vi "Calcul itératif.vi"(10 "Température capteur 1-2-3-4-Ambiant":dbl[](array[numeric]), 11 "Position des capteurs":dbl[][](array[numeric])) -> (3 "DATA - T/R1/R2/R3":dbl[](array[numeric]) format="%#_13g")   [LabVIEW 2018]
panel:
  in  "T max":dbl
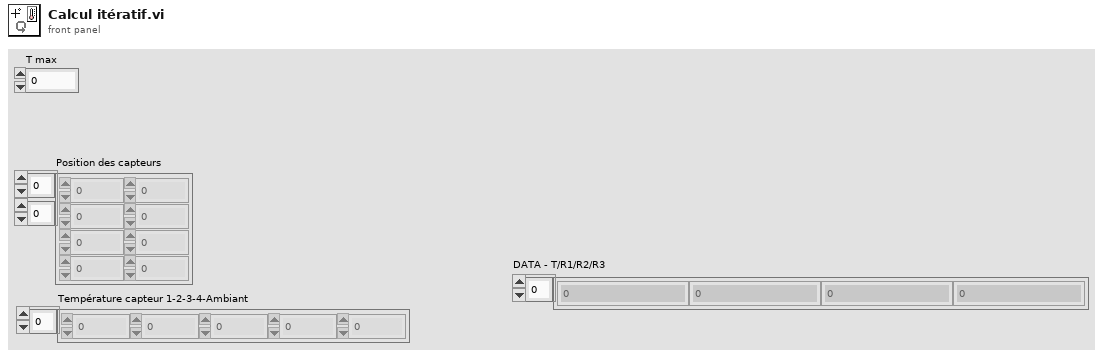
[diagram p1: front panel]
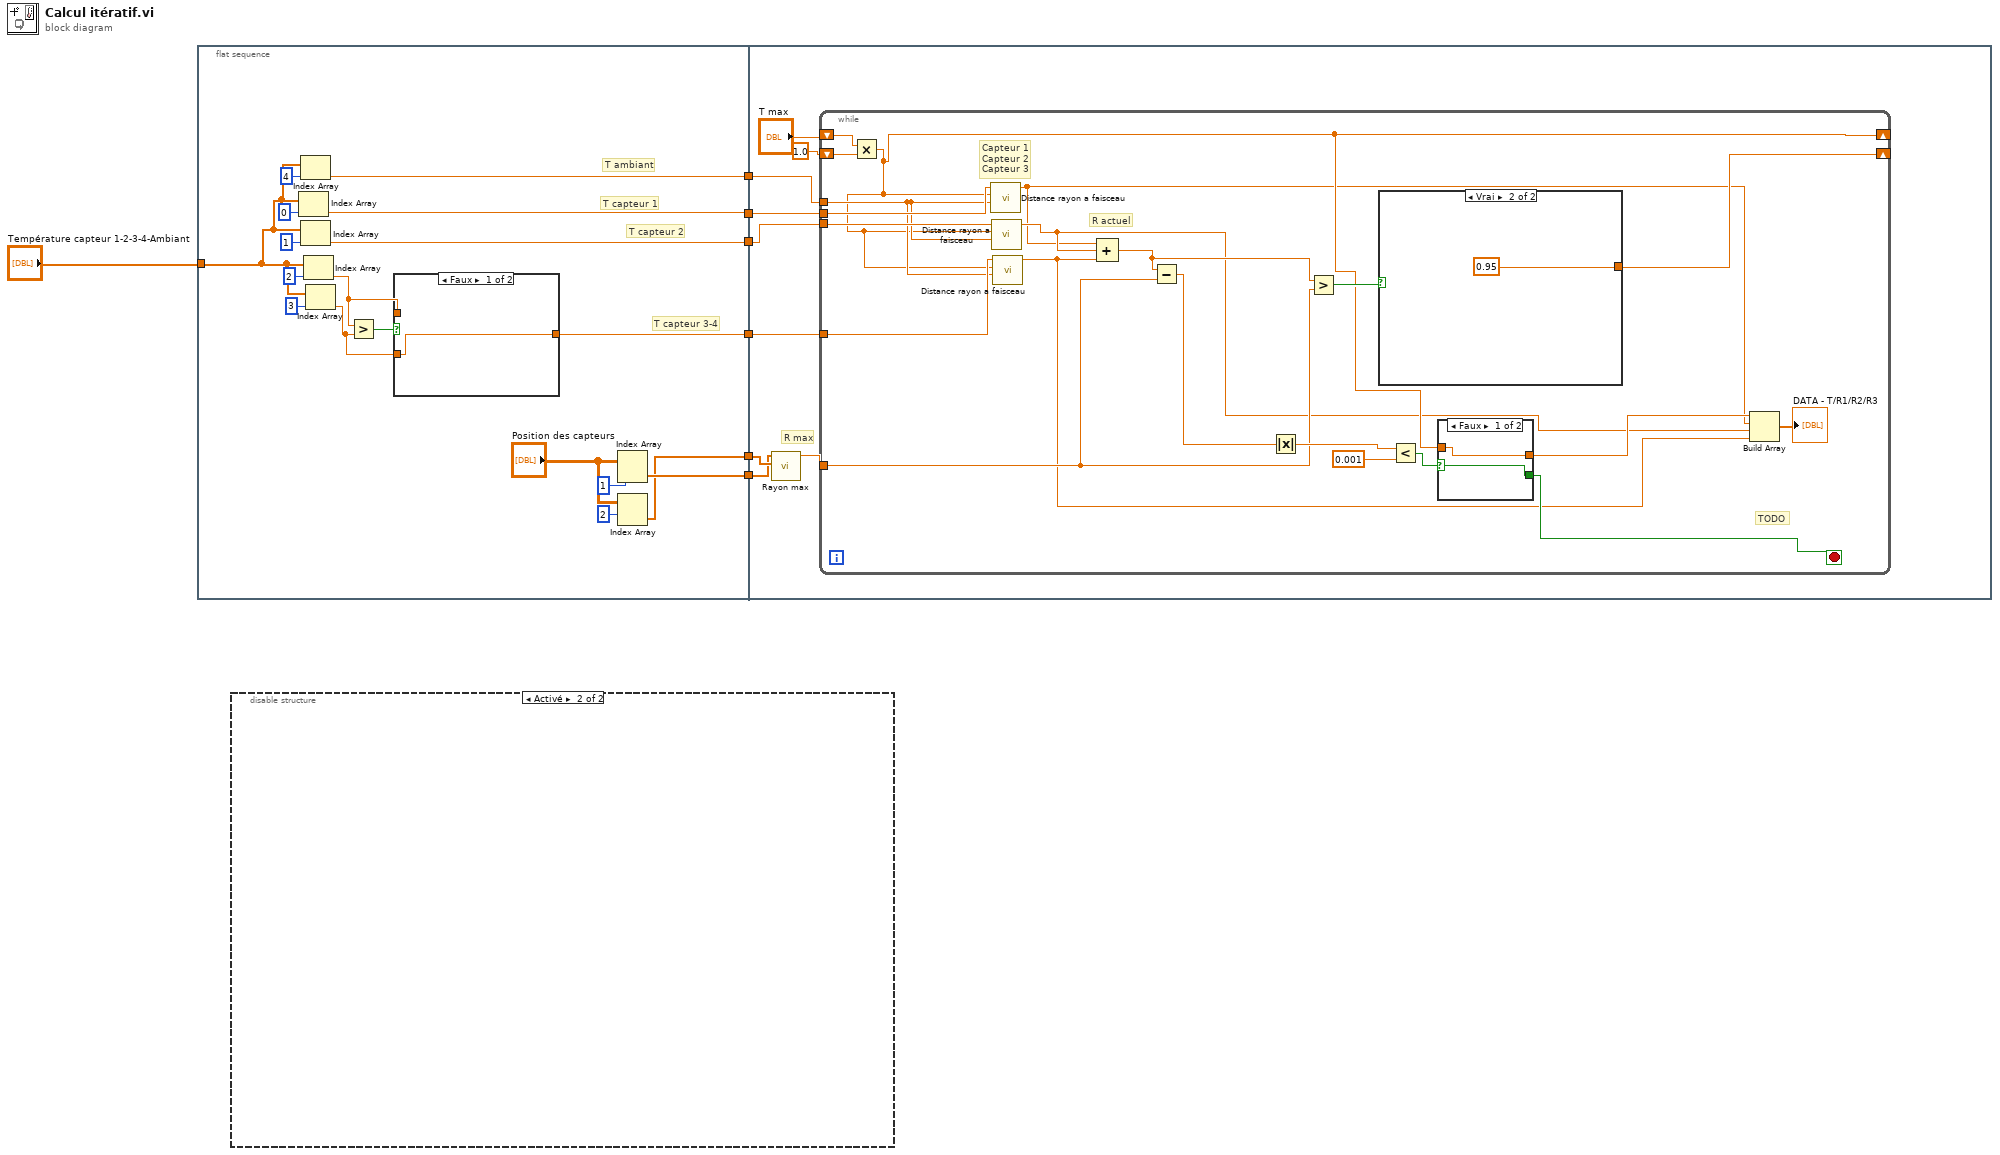
[diagram p0: block diagram]
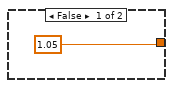
[diagram p4: hidden frame]
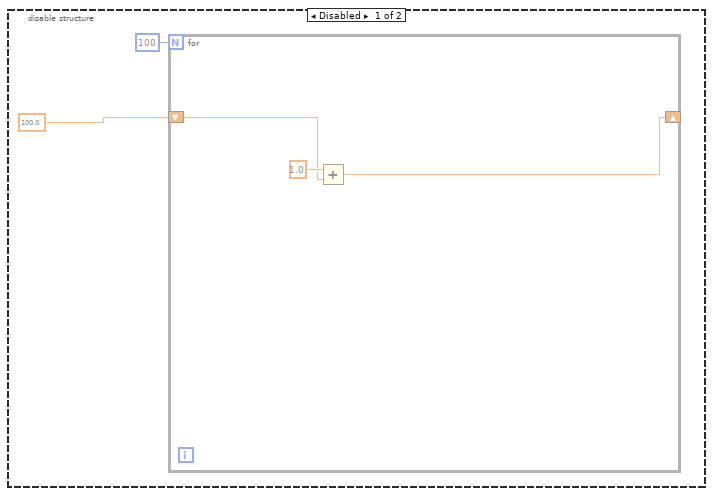
[diagram p5: hidden frame]
diagram:
  n1 = flat-sequence {
    tunnel: "Température capteur 1-2-3-4-Ambiant" -> [w15]
    tunnel: [w21] -> w7
    tunnel: [w17] -> w6
    tunnel: [w16] -> w5
    tunnel: [w13] -> w4
    tunnel: [w9] -> w2
    tunnel: [w8] -> w1
    tunnel: w7 -> [w33]
    tunnel: w6 -> [w36]
    tunnel: w5 -> [w34]
    tunnel: w4 -> [w35]
    tunnel: w2 -> [w29]
    tunnel: w1 -> [w30]
    frame #0 {
      # "T capteur 3-4"
      # "T capteur 2"
      # "T capteur 1"
      # "T ambiant"
      n2 = Index Array(array=w15, index=0 ("indice")) -> (element=w17:dbl)
      n3 = Index Array(array=w15, index=4 ("indice")) -> (element=w13:dbl)
      n4 = Index Array(array=w15, index=1 ("indice")) -> (element=w16:dbl)
      n5 = Index Array(array=w15, index=2 ("indice")) -> (element=w22:dbl)
      n6 = Index Array(array=w15, index=3 ("indice")) -> (element=w20:dbl)
      n7 = Greater?(x=w22, y=w20) -> (0:w23:bool)
      n8 = case shown="Faux" w23 {
        tunnel: [w26 w27] -> w21
        tunnel: w22 -> [_ w27]
        tunnel: w20 -> [w26 _]
        frame False {
        }
        frame True {
        }
      }
      n9 = Index Array(array="Position des capteurs", index (row)=1 ("indice (ligne)")) -> (element=w9:dbl[])  [unwired: 1 in]
      n10 = Index Array(array="Position des capteurs", index (row)=2 ("indice (ligne)")) -> (element=w8:dbl[])  [unwired: 1 in]
    }
    frame #1 {
      # "R max"
      n11 = call "Rayon max.vi"("Capteur 3 ou 4"=w30, "Capteur 2"=w29) -> ("Rayon max"=w28:dbl)  [unwired: 9 in]
      n12 = while {
        tunnel: w36 -> [w57]
        tunnel: w35 -> [w54]
        tunnel: w34 -> [w56]
        tunnel: w33 -> [w55]
        shift-right: [w51] -> _
        shift-left: 1.0 -> [w45]
        shift-right: [w42] -> _
        shift-left: "T max" -> [w44]
        tunnel: w28 -> [w43]
        stop <- w49 stop-if-true
        # "Capteur 1\nCapteur 2\nCapteur 3"
        # "R actuel"
        # "TODO"
        n13 = Multiply(x=w44, y=w45) -> (x*y=w42:dbl)
        n14 = call "Distance rayon a faisceau.vi"("T ambiant"=w54, "T max"=w42, "T capteur"=w57) -> ("Rayon"=w37:dbl)  [unwired: 8 in]
        n15 = call "Distance rayon a faisceau.vi"("T ambiant"=w54, "T max"=w42, "T capteur"=w56) -> ("Rayon"=w40:dbl)  [unwired: 8 in]
        n16 = call "Distance rayon a faisceau.vi"("T ambiant"=w54, "T max"=w42, "T capteur"=w55) -> ("Rayon"=w39:dbl)  [unwired: 8 in]
        n17 = Compound Arithmetic op=ADD(w37, w40, w39) -> (w52:dbl)
        n18 = Subtract(x=w52, y=w43) -> (x-y=w53:dbl)
        n19 = Absolute Value(x=w53) -> (abs(x)=w47:dbl)
        n20 = Greater?(x=w52, y=w43) -> (0:w50:bool)
        n21 = case shown="Vrai" w50 {
          tunnel: [1.05 0.95] -> w51
          frame False {
          }
          frame True {
          }
        }
        n22 = Less?(x=w47, y=0.001) -> (x < y?=w46:bool)
        n23 = case shown="Faux" w46 {
          selector: w46 -> [w59 w61]
          tunnel: [w59 w61] -> w49
          tunnel: w42 -> [w58 w60]
          tunnel: [w58 w60] -> w41
          frame False {
          }
          frame True {
          }
        }
        n24 = Build Array(w41, w37, w40, w39) -> (→"DATA - T/R1/R2/R3":dbl[])
      }
    }
  }
  n25 = disable-structure shown="Activé" {
    frame Disabled {
      n26 = for {
        N: 100 -> [_]
        shift-right: [w66] -> _
        shift-left: 100.0 -> [w67]
        n27 = Add(x=1.0, y=w67) -> (x+y=w66:dbl)
      }
    }
    frame Enabled {
    }
  }
